vi "Add Pre Section.vi"(5 "no of points":u8, 6 "Identifier":u32, 7 "WheelID (if need)":u8, 8 "error in (no error)":errorcluster, 11 "Item Ref in":T1=18446744073709551615 format="%.0x") -> (0 "error out":errorcluster, 3 "Item Ref out":T1=18446744073709551615 format="%.0x", 4 "adv para":i32)   [LabVIEW 2023, in "Vires VTD System Explorer.lvlib"]
uses:
  Vires VTD System Explorer.lvlib
  <vilib>/NI VeriStand/Custom Device API/Custom Device Item Ref.ctl
  Shared/Constants.vi
  <vilib>/NI VeriStand/Custom Device API/Custom Device API.lvlib
  Shared/Vires VTD Shared.lvlib
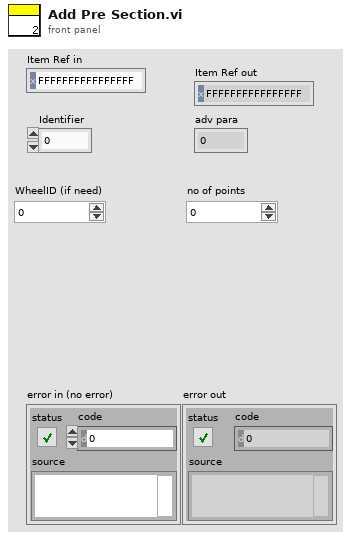
[diagram p1: front panel]
types:
  T1 = typedef "Custom Device API.lvlib/Custom Device Item Ref.ctl" = u64
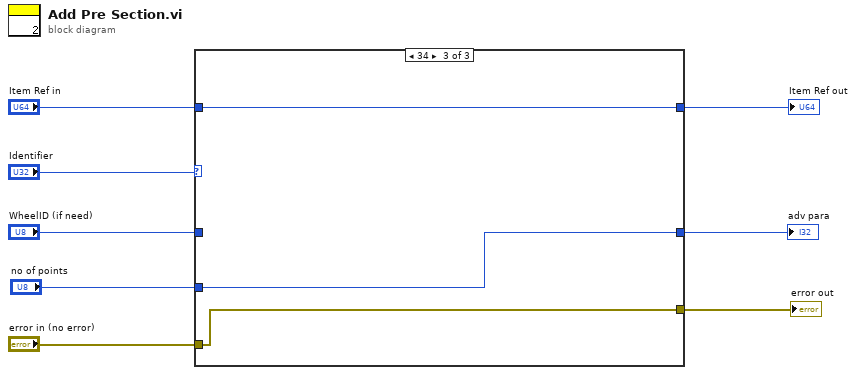
[diagram p0: block diagram]
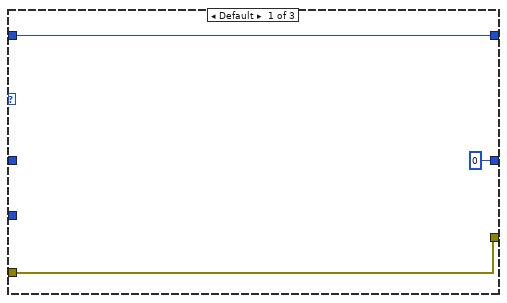
[diagram p2: hidden frame]
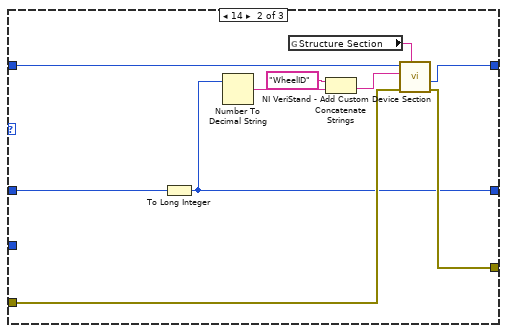
[diagram p3: hidden frame]
diagram:
  n1 = case shown="34" "Identifier" {
    tunnel: "Item Ref in" -> [w11 w21 w24]
    tunnel: [w11 w20 w24] -> w6
    tunnel: "error in (no error)" -> [w10 w18 w22]
    tunnel: [w10 w19 w22] -> w4
    tunnel: [0 w14 w23] -> w3
    tunnel: "WheelID (if need)" -> [_ w12 _]
    tunnel: "no of points" -> [_ _ w23]
    frame Default {
    }
    frame 14 {
      n2 = To Long Integer(number=w12) -> (32bit integer=w14:i32)
      n3 = Number To Decimal String(number=w14) -> (decimal integer string=w16:string)  [unwired: 1 in]
      n4 = global read "Constants.vi" "Structure Section"() -> (w13:string)
      n5 = Concatenate Strings("WheelID" ("string"), w16) -> (w15:string)
      n6 = call <vilib>:"NI VeriStand - Add Custom Device Section.vi"("GUID (Default Section)"=w13, "error in (no error)"=w18, "Section Name"=w15, "Parent Ref in"=w21) -> ("error out"=w19:errorcluster, "Section Ptr"=w20:T1)  [unwired: 4 in, 2 out]
    }
    frame 34 {
    }
  }
  "error out" <- w4
  "Item Ref out" <- w6
  "adv para" <- w3
